vi "Open Connection.vi"(8 "error in":errorcluster, 10 "password":string, 11 "username":string) -> (0 "error out":errorcluster, 3 "Spark Reference":T1)   [LabVIEW 2014, in "Spark API.lvlib"]
uses:
  Spark API.lvlib
  Controls/Spark Reference.ctl
  <vilib>/httpClient/ClientHandle.ctl
  Controls/Device Query JSON.ctl
  Controls/Devices Query JSON.ctl
  <vilib>/httpClient/LabVIEWHTTPClient.lvlib
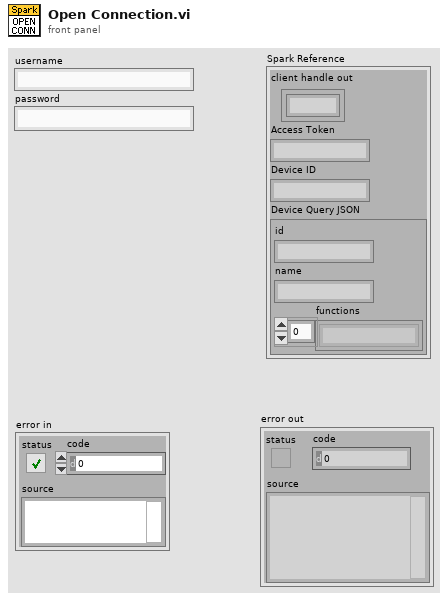
[diagram p1: front panel]
types:
  T1 = typedef "Spark API.lvlib/Spark Reference.ctl" = cluster{"client handle out":T2, "Access Token":string, "Device ID":string, "Device Query JSON":T3}
  T2 = typedef "LabVIEWHTTPClient.lvlib/ClientHandle.ctl" = refnum<k1>
  T3 = typedef "Spark API.lvlib/Device Query JSON.ctl" = cluster{"id":string, "name":string, "functions":string[]}
  T4 = typedef "Spark API.lvlib/Devices Query JSON.ctl" = cluster{"id":string, "name":string, "connected":bool}[]
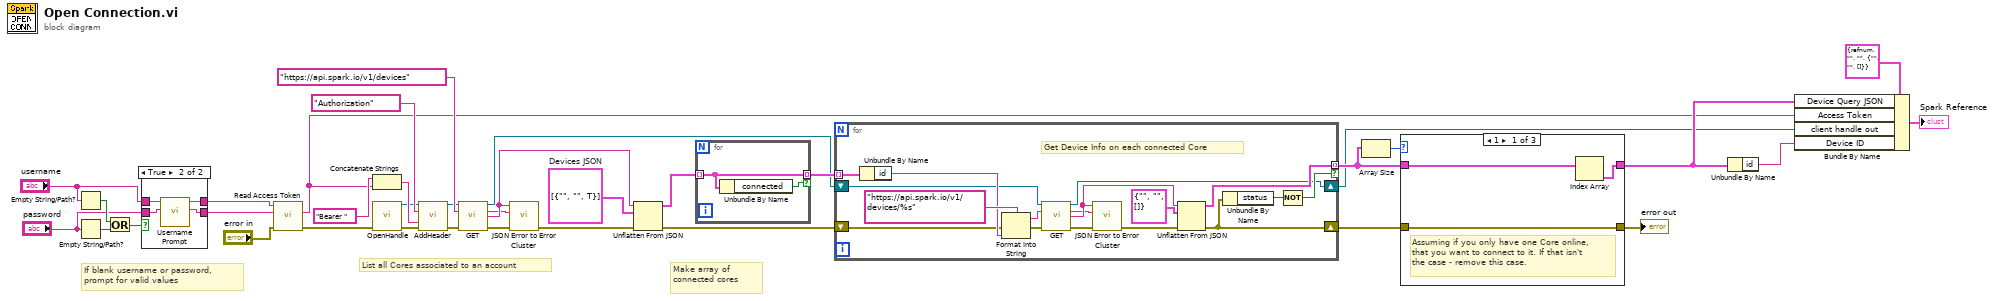
[diagram p0: block diagram]
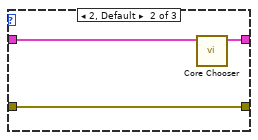
[diagram p3: hidden frame]
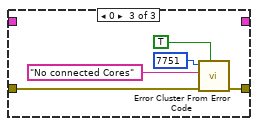
[diagram p4: hidden frame]
diagram:
  w33 = T4 [{"id"="", "name"="", "connected"=TRUE}]  # Devices JSON
  # "Make array of connected cores"
  # "If blank username or password, prompt for valid values"
  # "List all Cores associated to an account"
  n1 = Empty String/Path?(string/path="username") -> (empty?=w18:bool)
  n2 = Empty String/Path?(string/path="password") -> (empty?=w17:bool)
  n3 = Or(x=w18, y=w17) -> (x .or. y?=w16:bool)
  n4 = case shown="True" w16 {
    tunnel: "username" -> [w38 w42]
    tunnel: "password" -> [w37 w41]
    tunnel: [w38 w40] -> w13
    tunnel: [w37 w39] -> w12
    frame False {
    }
    frame True {
      n5 = call "Username Prompt.vi"("Password"=w41, "Username"=w42) -> ("Password out"=w39:string, "Username out"=w40:string)  [unwired: 8 in]
    }
  }
  n6 = call "Read Access Token.vi"("error in"="error in", "password"=w12, "username"=w13) -> ("error out"=w5:errorcluster, "token"=w1:string)  [unwired: 7 in]
  n7 = Concatenate Strings("Bearer " ("string"), w1) -> (w9:string)
  n8 = call <vilib>:"OpenHandle.vi"("error in (no error)"=w5) -> ("client handle out"=w6:T2, "error out"=w7:errorcluster)  [unwired: 13 in]
  n9 = call <vilib>:"AddHeader.vi"("client handle"=w6, "header"="Authorization", "value"=w9, "error in (no error)"=w7) -> ("client handle out"=w3:T2, "error out"=w4:errorcluster)  [unwired: 10 in]
  n10 = call <vilib>:"GET.vi"("client handle"=w3, "url"="https://api.spark.io/v1/devices", "error in (no error)"=w4) -> ("client handle out"=w24:T2, "headers"=w19:string, "body"=w20:string, "error out"=w22:errorcluster)  [unwired: 9 in]
  n11 = call "JSON Error to Error Cluster.vi"("error in (no error)"=w22, "headers"=w19, "JSON string"=w20) -> ("error out"=w21:errorcluster)  [unwired: 8 in]
  n12 = Unflatten From JSON(JSON string=w20, type and defaults=w33, error in (no error)=w21) -> (value=w32:T4, error out=w23:errorcluster)  [unwired: 4 in]
  n13 = for {
    tunnel: w32 -> [w44] mode=indexing
    tunnel: [w44] -> w30 mode=indexing if=w43
    n14 = Unbundle By Name(w44) -> ("connected"=w43:bool)
  }
  n15 = for {
    tunnel: w30 -> [w58] mode=indexing
    shift-right: [w51] -> w29
    shift-left: w23 -> [w55]
    tunnel: [w54] -> w28 mode=indexing if=w52
    shift-right: [w50] -> w2
    shift-left: w24 -> [w49]
    # "Get Device Info on each connected Core"
    n16 = Unbundle By Name(w58) -> ("id"=w57:string)
    n17 = Format Into String(format string="https://api.spark.io/v1/devices/%s" ("url"), error in=w55, w57) -> (resulting string=w60:string, error out=w61:errorcluster)  [unwired: 1 in]
    n18 = call <vilib>:"GET.vi"("client handle"=w49, "url"=w60, "error in (no error)"=w61) -> ("client handle out"=w50:T2, "headers"=w45:string, "body"=w46:string, "error out"=w48:errorcluster)  [unwired: 9 in]
    n19 = call "JSON Error to Error Cluster.vi"("error in (no error)"=w48, "headers"=w45, "JSON string"=w46) -> ("error out"=w47:errorcluster)  [unwired: 8 in]
    n20 = Unflatten From JSON(JSON string=w46, type and defaults=T3 {"id"="", "name"="", "functions"=[]} ("Device Query JSON"), error in (no error)=w47) -> (value=w54:T3, error out=w51:errorcluster)  [unwired: 4 in]
    n21 = Unbundle By Name(w51) -> ("status"=w53:bool)
    n22 = Not(x=w53) -> (.not. x?=w52:bool)
  }
  n23 = Array Size(array=w28) -> (size(s)=w31:i32)
  n24 = case shown="1" w31 {
    tunnel: w29 -> [w62 w67 w69]
    tunnel: w28 -> [w64 w65 _]
    tunnel: [w63 w66 _] -> w26
    tunnel: [w62 w67 w68] -> w27
    frame 1 {
      # "Assuming if you only have one Core online, that you want to connect to it. If that isn't the case - remove this case."
      n25 = Index Array(array=w64) -> (element=w63:T3)  [unwired: 1 in]
    }
    frame 2, Default {
      n26 = call "Core Chooser.vi"("Online Cores"=w65) -> ("Selectied Core"=w66:T3)  [unwired: 10 in]
    }
    frame 0 {
      n27 = call <vilib>:"Error Cluster From Error Code.vi"("show call chain? (False)"=TRUE, "error in (no error)"=w69, "error message (\"\")"="No connected Cores" ("error message (\"\")"), "error code (0)"=7751) -> ("error out"=w68:errorcluster)  [unwired: 5 in]
    }
  }
  "error out" <- w27
  n28 = Unbundle By Name(w26) -> ("id"=w25:string)
  n29 = Bundle By Name(cluster=T1 {"client handle out"=refnum, "Access Token"="", "Device ID"="", "Device Query JSON"={"id"="", "name"="", "functions"=[]}} ("Spark Reference"), "Device Query JSON"=w26, "Access Token"=w1, "client handle out"=w2, "Device ID"=w25) -> (→"Spark Reference":T1)
